vi "HiTechnic SMUX Read_DM.vi"(6 "Offset":u8, 7 "Port":T2 items=["Port 1", "Port 2", "Port 3", "Port 4"], 8 "Parameters":u8[](array[numeric])=[0, 0, 0, 0, 0] format="%x", 9 "Read Length":u8, 10 "MUX Port":u8, 11 "NXT/EV3":T1) -> (0 "Success?":bool, 2 "Array":u8[](array[numeric]), 3 "NXT/EV3":T1 caption="NXT")   [LabVIEW 2012]
doc: "Reads the Sensor Multiplexer to retrieve data from the selected sensor."
uses:
  <vilib>/NXT/Block Support/NXT_InputPort.ctl
  <vilib>/NXT/Subs/LVHSConnector.ctl
  <vilib>/NXT/LegoClasses/BrickReference/BrickReference.lvclass
  <vilib>/NXT/Block Support/HWPage.SensorType.ctl
  <vilib>/NXT/Block Support/HWPage.SensorMode.ctl
panel:
  in  "MUX Port Mode":u8[](array[numeric])=[0, 0, 0, 0]
  # "Variables"
  # "MUX Port Mode, once initialized, will keep\nthe mode byte of each possible MUX port.\nIndex is Port * 4 + (MUX Port -1)."
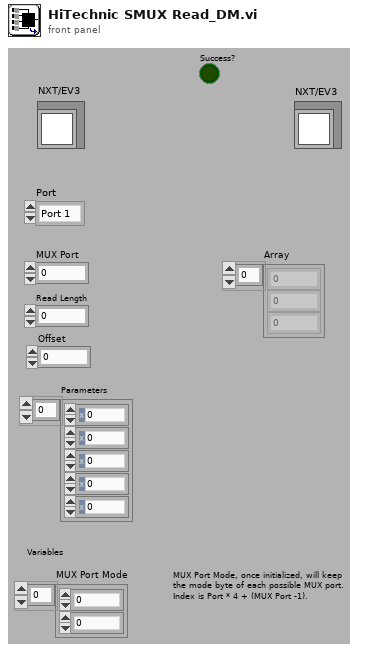
[diagram p1: front panel]
types:
  T1 = typedef "LVHSConnector.ctl" = refnum<class "BrickReference.lvclass">
  T2 = typedef "NXT_InputPort.ctl" = u32
  T3 = typedef "HWPage.SensorType.ctl" = u8
  T4 = typedef "HWPage.SensorMode.ctl" = u8
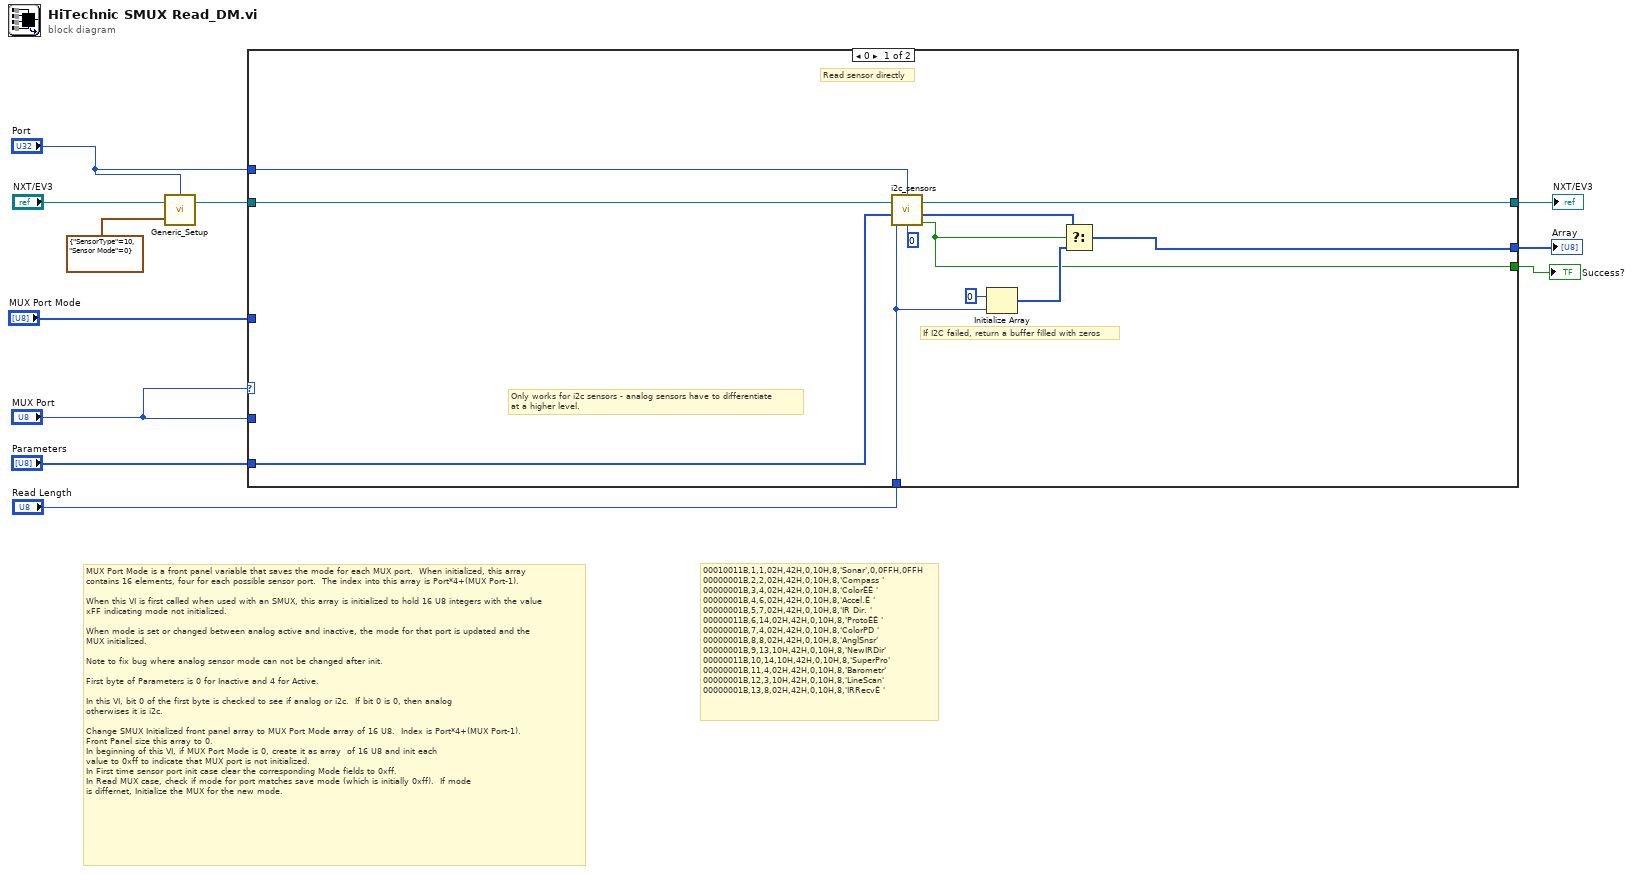
[diagram p0: block diagram]
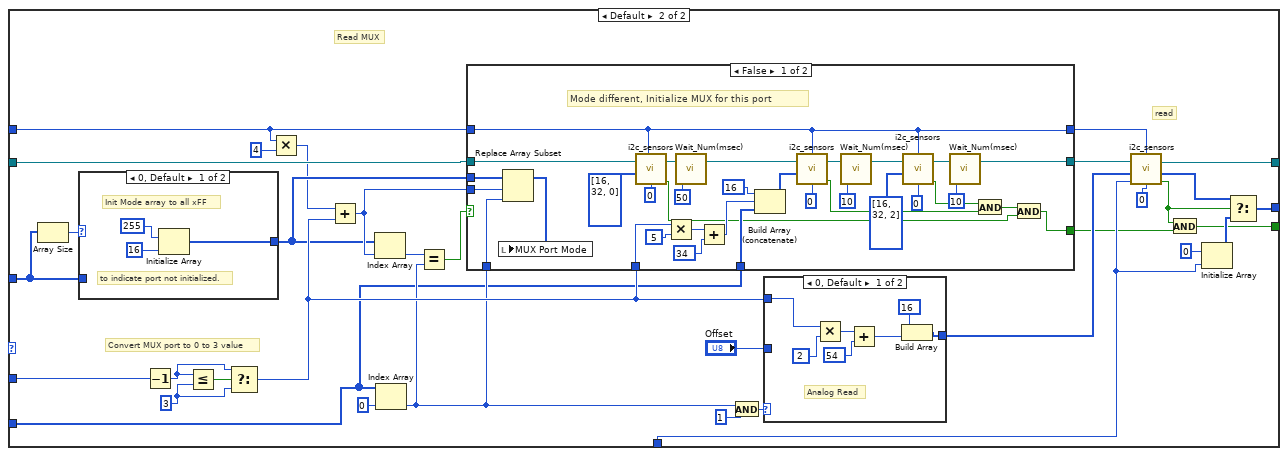
[diagram p2: hidden frame]
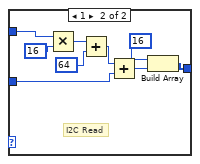
[diagram p4: hidden frame]
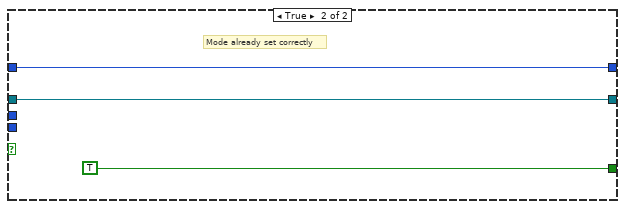
[diagram p5: hidden frame]
diagram:
  # "MUX Port Mode is a front panel variable that saves the mode for each MUX port.  When initialized, this array\ncontains 16 elements, four for each possible sensor port.  The index into this array is Port*4+(MUX Port-1).\n\nWhen this VI is first called when used with an SMUX, this array is initialized to hold 16 U8 integers with the value\nxFF indicating mode not initialized.\n\nWhen mode is set or changed between analog active and inactive, the mode for that port is updated and the\nMUX initialized.\n\nNote to fix bug where analog sensor mode can not be changed after init.\n\nFirst byte of Parameters is 0 for Inactive and 4 for Active.\n\nIn this VI, bit 0 of the first byte is checked to see if analog or i2c.  If bit 0 is 0, then analog\notherwises it is i2c.\n\nChange SMUX Initialized front panel array to MUX Port Mode array of 16 U8.  Index is Port*4+(MUX Port-1).\nFront Panel size this array to 0.\nIn beginning of this VI, if MUX Port Mode is 0, create it as array  of 16 U8 and init each\nvalue to 0xff to indicate that MUX port is not initialized.\nIn First time sensor port init case clear the corresponding Mode fields to 0xff.\nIn Read MUX case, check if mode for port matches save mode (which is initially 0xff).  If mode\nis differnet, Initialize the MUX for the new mode."
  # "00010011B,1,1,02H,42H,0,10H,8,'Sonar',0,0FFH,0FFH\n00000001B,2,2,02H,42H,0,10H,8,'Compass '\n00000001B,3,4,02H,42H,0,10H,8,'ColorÊÊ '\n00000001B,4,6,02H,42H,0,10H,8,'Accel.Ê '\n00000001B,5,7,02H,42H,0,10H,8,'IR Dir. '\n00000011B,6,14,02H,42H,0,10H,8,'ProtoÊÊ '\n00000001B,7,4,02H,42H,0,10H,8,'ColorPD '\n00000001B,8,8,02H,42H,0,10H,8,'AnglSnsr'\n00000001B,9,13,10H,42H,0,10H,8,'NewIRDir'\n00000011B,10,14,10H,42H,0,10H,8,'SuperPro'\n00000001B,11,4,02H,42H,0,10H,8,'Barometr'\n00000001B,12,3,10H,42H,0,10H,8,'LineScan'\n00000001B,13,8,02H,42H,0,10H,8,'IRRecvÊ '"
  n1 = call <vilib>:"Generic_Setup.vi"("Sensor Setup"=cluster{"SensorType":T3, "Sensor Mode":T4} {"SensorType"=10, "Sensor Mode"=0}, "NXT/EV3"="NXT/EV3", "Port"="Port") -> ("NXT/EV3"=w3:T1)  [unwired: 1 out]
  n2 = case shown="0" "MUX Port" {
    tunnel: [w13 w42] -> w11
    tunnel: "Port" -> [w14 w30]
    tunnel: "Parameters" -> [w22 w26]
    tunnel: "MUX Port" -> [_ w56]
    tunnel: w3 -> [w18 w28]
    tunnel: [w21 w55] -> w5
    tunnel: "Read Length" -> [w17 w40]
    tunnel: "MUX Port Mode" -> [_ w31]
    tunnel: [w12 w23] -> w1
    frame 0 {
      # "If I2C failed, return a buffer filled with zeros"
      # "Only works for i2c sensors - analog sensors have to differentiate \nat a higher level."
      # "Read sensor directly"
      n3 = call <vilib>:"i2c_sensors.vi"("Return Length"=w17, "Bytes to Write"=w22, "Wait (msec)"=u32 0, "NXT/EV3"=w18, "Port"=w14) -> ("Success?"=w12:bool, "Bytes read"=w19:u8[], "NXT/EV3"=w21:T1)
      n4 = Initialize Array(u8 0 ("element"), w17) -> (w15:u8[])
      n5 = Select(t=w19, s=w12, f=w15) -> (s? t:f=w13:u8[])
    }
    frame Default {
      w52 = u8 3 ("y")
      # "Convert MUX port to 0 to 3 value"
      # "read"
      # "Read MUX"
      n6 = Array Size(array=w31) -> (size(s)=w32:i32)
      n7 = case shown="0, Default" w32 {
        tunnel: w31 -> [_ w60]
        tunnel: [w57 w60] -> w29
        frame 0, Default {
          # "to indicate port not initialized."
          # "Init Mode array to all xFF"
          n8 = Initialize Array(u8 255, 16 ("dimension size")) -> (w57:u8[])
        }
        frame 16 {
          # "Port array already initialized."
        }
      }
      n9 = Decrement(x=w56) -> (x-1=w53:u8)
      n10 = Less Or Equal?(x=w53, y=w52) -> (x <= y?=w54:bool)
      n11 = Select(t=w53, s=w54, f=w52) -> (s? t:f=w37:u8)
      n12 = Multiply(x=w30, y=u8 4) -> (x*y=w27:T2)
      n13 = Add(x=w27, y=w37) -> (x+y=w34:T2)
      n14 = Index Array(array=w29, index=w34) -> (element=w36:u8)
      n15 = Index Array(array=w26, index=0) -> (element=w33:u8)
      n16 = Equal?(x=w36, y=w33) -> (x = y?=w35:bool)
      n17 = case shown="False" w35 {
        tunnel: w28 -> [w88 w111]
        tunnel: w30 -> [w86 w112]
        tunnel: w26 -> [w100 _]
        tunnel: [w89 w111] -> w39
        tunnel: [w86 w112] -> w45
        tunnel: w37 -> [w83 _]
        tunnel: w29 -> [w87 _]
        tunnel: w34 -> [w84 _]
        tunnel: w33 -> [w82 _]
        tunnel: [w77 TRUE] -> w24
        frame False {
          # "Mode different, Initialize MUX for this port"
          n18 = Replace Array Subset(array=w87, new element=w82, index=w84) -> (w85:u8[])
          n19 = local write "MUX Port Mode"(w85) -> ()
          n20 = call <vilib>:"i2c_sensors.vi"("Bytes to Write"=u8[] [16, 32, 0], "Wait (msec)"=u32 0, "NXT/EV3"=w88, "Port"=w86) -> ("Success?"=w78:bool, "NXT/EV3"=w96:T1)  [unwired: 1 in, 1 out]
          n21 = Multiply(x=w83, y=u8 5 ("ReturnLength")) -> (x*y=w103:u8)
          n22 = call <vilib>:"Wait_Num(msec).vi"("Time (100 msec)"=u32 50, "NXT/EV3"=w96) -> ("NXT/EV3"=w95:T1)  [unwired: 2 in]
          n23 = Add(x=w103, y=u8 34) -> (x+y=w101:u8)
          n24 = Build Array (concatenate)(u8 16, w101, w100) -> (w99:u8[])
          n25 = call <vilib>:"i2c_sensors.vi"("Bytes to Write"=w99, "Wait (msec)"=u32 0, "NXT/EV3"=w95, "Port"=w86) -> ("Success?"=w80:bool, "NXT/EV3"=w93:T1)  [unwired: 1 in, 1 out]
          n26 = call <vilib>:"Wait_Num(msec).vi"("Time (100 msec)"=u32 10, "NXT/EV3"=w93) -> ("NXT/EV3"=w92:T1)  [unwired: 2 in]
          n27 = call <vilib>:"i2c_sensors.vi"("Bytes to Write"=u8[] [16, 32, 2], "Wait (msec)"=u32 0, "NXT/EV3"=w92, "Port"=w86) -> ("Success?"=w81:bool, "NXT/EV3"=w90:T1)  [unwired: 1 in, 1 out]
          n28 = call <vilib>:"Wait_Num(msec).vi"("Time (100 msec)"=u32 10, "NXT/EV3"=w90) -> ("NXT/EV3"=w89:T1)  [unwired: 2 in]
          n29 = And(x=w81, y=w80) -> (x .and. y?=w79:bool)
          n30 = And(x=w79, y=w78) -> (x .and. y?=w77:bool)
        }
        frame True {
          # "Mode already set correctly"
        }
      }
      n31 = And(x=w33, y=u8 1) -> (x .and. y?=w50:u8)
      n32 = case shown="0, Default" w50 {
        tunnel: w37 -> [w62 w72]
        tunnel: "Offset" -> [_ w70]
        tunnel: [w61 w68] -> w48
        frame 0, Default {
          # "Analog Read"
          n33 = Multiply(x=w62, y=u8 2 ("ReturnLength")) -> (x*y=w64:u8)
          n34 = Add(x=w64, y=u8 54) -> (x+y=w67:u8)
          n35 = Build Array(u8 16, w67) -> (w61:u8[])
        }
        frame 1 {
          # "I2C Read"
          n36 = Multiply(x=w72, y=u8 16 ("ReturnLength")) -> (x*y=w75:u8)
          n37 = Add(x=w75, y=u8 64) -> (x+y=w71:u8)
          n38 = Add(x=w71, y=w70) -> (x+y=w69:u8)
          n39 = Build Array(u8 16, w69) -> (w68:u8[])
        }
      }
      n40 = call <vilib>:"i2c_sensors.vi"("Return Length"=w40, "Bytes to Write"=w48, "Wait (msec)"=u32 0, "NXT/EV3"=w39, "Port"=w45) -> ("Success?"=w25:bool, "Bytes read"=w41:u8[], "NXT/EV3"=w55:T1)
      n41 = And(x=w25, y=w24) -> (x .and. y?=w23:bool)
      n42 = Initialize Array(u8 0 ("element"), w40) -> (w43:u8[])
      n43 = Select(t=w41, s=w25, f=w43) -> (s? t:f=w42:u8[])
    }
  }
  "Array" <- w11
  "NXT/EV3" <- w5
  "Success?" <- w1
